vi "test json to variant string.vi"(8 "error in (no error)":errorcluster) -> (0 "error out":errorcluster)   [LabVIEW 2019, in "labview_json_tests.lvlib"]
uses:
  labview_json_tests.lvlib
  lib/labview_json.lvlib
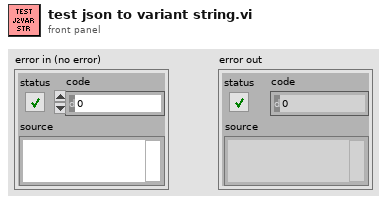
[diagram p1: front panel]
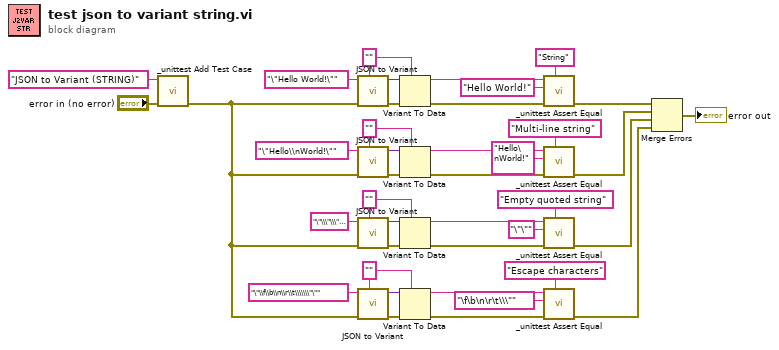
[diagram p0: block diagram]
diagram:
  w8 = ""
  w7 = ""
  w6 = ""
  w5 = ""
  n1 = call "_unittest Add Test Case.vi"("error in (no error)"="error in (no error)", "Test Case"="JSON to Variant (STRING)") -> ("error out"=w21:errorcluster)  [unwired: 9 in]
  n2 = call "JSON to Variant.vi"("Variant Type"=w5, "error in (no error)"=w21, "JSON"="\"Hello World!\"") -> ("error out"=w26:errorcluster, "Variant out"=w12:variant)  [unwired: 7 in]
  n3 = call "JSON to Variant.vi"("Variant Type"=w6, "error in (no error)"=w21, "JSON"="\"Hello\\nWorld!\"") -> ("error out"=w24:errorcluster, "Variant out"=w11:variant)  [unwired: 7 in]
  n4 = call "JSON to Variant.vi"("Variant Type"=w7, "error in (no error)"=w21, "JSON"="\"\\\"\\\"\"") -> ("error out"=w23:errorcluster, "Variant out"=w10:variant)  [unwired: 7 in]
  n5 = call "JSON to Variant.vi"("Variant Type"=w8, "error in (no error)"=w21, "JSON"="\"\\f\\b\\n\\r\\t\\\\\\\"\"") -> ("error out"=w22:errorcluster, "Variant out"=w9:variant)  [unwired: 7 in]
  n6 = Variant To Data(error in=w26, type=w5, Variant=w12) -> (data=w4:string, error out=w16:errorcluster)
  n7 = Variant To Data(error in=w24, type=w6, Variant=w11) -> (data=w3:string, error out=w15:errorcluster)
  n8 = Variant To Data(error in=w23, type=w7, Variant=w10) -> (data=w2:string, error out=w14:errorcluster)
  n9 = Variant To Data(error in=w22, type=w8, Variant=w9) -> (data=w1:string, error out=w13:errorcluster)
  n10 = call "_unittest Assert Equal.vi"("Message"="String", "error in (no error)"=w16, "Expected Value"="Hello World!", "Actual Value"=w4) -> ("error out"=w38:errorcluster)  [unwired: 7 in]
  n11 = call "_unittest Assert Equal.vi"("Message"="Multi-line string", "error in (no error)"=w15, "Expected Value"="Hello\nWorld!", "Actual Value"=w3) -> ("error out"=w35:errorcluster)  [unwired: 7 in]
  n12 = call "_unittest Assert Equal.vi"("Message"="Empty quoted string", "error in (no error)"=w14, "Expected Value"="\"\"", "Actual Value"=w2) -> ("error out"=w32:errorcluster)  [unwired: 7 in]
  n13 = call "_unittest Assert Equal.vi"("Message"="Escape characters", "error in (no error)"=w13, "Expected Value"="\f\b\n\r\t\\\"", "Actual Value"=w1) -> ("error out"=w31:errorcluster)  [unwired: 7 in]
  n14 = Merge Errors(w38, w35, w32, w31) -> (→"error out":errorcluster)
